vi "DIScope Globals.vi"() -> ()   [LabVIEW 2015, in "ECS-RT.lvlib"]
uses:
  ECS-RT.lvlib
panel:
  out "DI4ScopeRunning":bool
  out "DI3ScopeRunning":bool
  out "DI2ScopeRunning":bool
  out "DI1ScopeRunning":bool
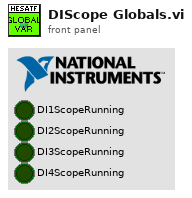
[diagram p1: front panel]
diagram:
